vi "readI8.vi"(8 "error in (no error)":errorcluster, 11 "ModbusBuffer in":refnum<class "ModbusBuffer.lvclass">) -> (0 "error out":errorcluster, 2 "Output":i8, 3 "ModbusBuffer out":refnum<class "ModbusBuffer.lvclass">)   [LabVIEW 2016, in "RTModbus.lvlib" / "ModbusBuffer.lvclass"]
uses:
  ModbusBuffer.lvclass
  ModbusBuffer.lvclass/ModbusBuffer.ctl
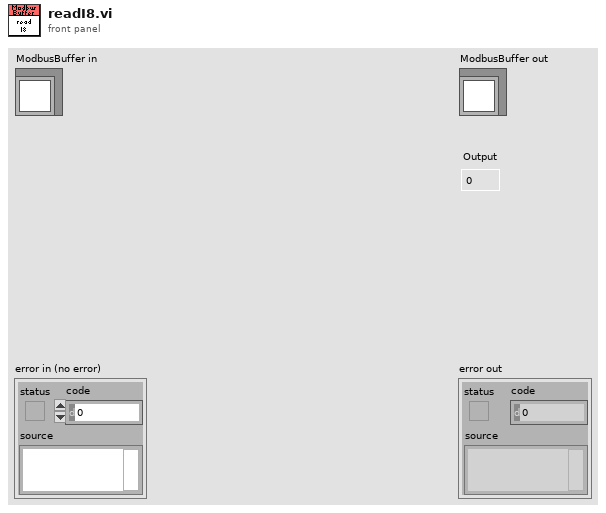
[diagram p1: front panel]
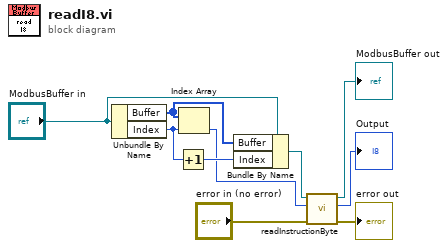
[diagram p0: block diagram]
diagram:
  n1 = Unbundle By Name("ModbusBuffer in") -> ("Buffer"=w8:u16[], "Index"=w7:i32)
  n2 = Increment(x=w7) -> (x+1=w9:i32)
  n3 = Index Array(array=w8, index=w7) -> (element=w6:u16)
  n4 = Bundle By Name(cluster="ModbusBuffer in", "Buffer"=w8, "Index"=w9) -> (w5:refnum<class "ModbusBuffer.lvclass">)
  n5 = call "readInstructionByte.vi"("error in (no error)"="error in (no error)", "Instruction"=w6, "ModbusBuffer in"=w5) -> ("error out"=→"error out":errorcluster, "Output"=→"Output":u8, "ModbusBuffer out"=→"ModbusBuffer out":refnum<class "ModbusBuffer.lvclass">)  [unwired: 6 in]
